vi "FV_stop_motion.vi"(8 "error in":errorcluster, 11 "VISA in":refnum<visa-resource-name>) -> (0 "error out":errorcluster, 1 "status":bool, 3 "VISA out":refnum<visa-resource-name>)   [LabVIEW 2019]
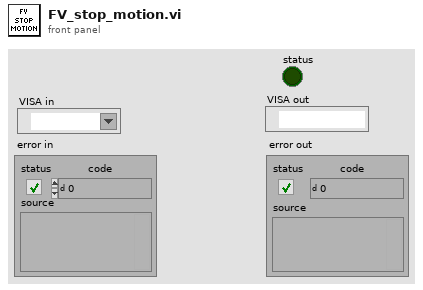
[diagram p1: front panel]
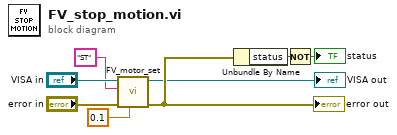
[diagram p0: block diagram]
diagram:
  n1 = call "FV_motor_set.vi"("delay  (sec)"=0.1, "error in"="error in", "command"="ST", "VISA in"="VISA in") -> ("error out"=w2:errorcluster, "VISA out"=→"VISA out":refnum<visa-resource-name>)  [unwired: 6 in]
  "error out" <- w2
  n2 = Unbundle By Name(w2) -> ("status"=w5:bool)
  n3 = Not(x=w5) -> (.not. x?=→"status":bool)
